vi "json Parse I32 - array path.vi"(8 "error in (no error)":errorcluster, 9 "default":i32, 10 "path":string[](array[string]), 11 "JSON Document in":refnum<class "JSON Document.lvclass">) -> (0 "error out":errorcluster, 1 "defaulted?":bool, 2 "value":i32, 3 "JSON Document out":refnum<class "JSON Document.lvclass">)   [LabVIEW 2015, in "JSON Document.lvclass"]
uses:
  JSON Document.lvclass
  json Parse I32 - string path.vi
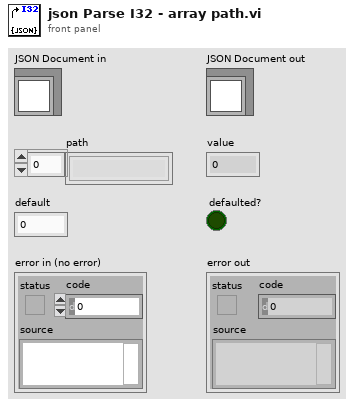
[diagram p1: front panel]
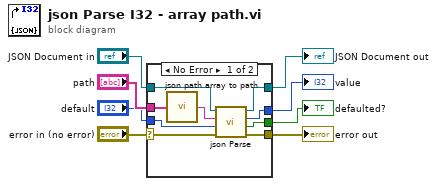
[diagram p0: block diagram]
diagram:
  n1 = case shown="No Error" "error in (no error)" {
    selector: "error in (no error)" -> [w10 w20]
    tunnel: [w11 w20] -> w4
    tunnel: [w13 w19] -> w2
    tunnel: "JSON Document in" -> [w17 w19]
    tunnel: "default" -> [w14 w18]
    tunnel: "path" -> [w16 _]
    tunnel: [w12 w18] -> w3
    tunnel: [w9 _] -> w1
    frame No Error {
      n2 = call "json path array to path.vi"("path"=w16) -> ("String"=w15:string)
      n3 = call-poly "json Parse.vi"("error in (no error)"=w10, "default"=w14, "path"=w15, "JSON Document in"=w17) -> ("error out"=w11:errorcluster, "defaulted?"=w9:bool, "value"=w12:i32, "JSON Document out"=w13:refnum<class "JSON Document.lvclass">)  [unwired: 4 in]
    }
    frame Error {
    }
  }
  "error out" <- w4
  "JSON Document out" <- w2
  "value" <- w3
  "defaulted?" <- w1
